vi "example_01_authorization.vi"() -> ()   [LabVIEW 2015, in "lv-dropbox.lvlib"]
uses:
  lv-dropbox.lvlib
  <vilib>/Platform/browser.llb/Open URL in Default Browser (string).vi
panel:
  in  "access_code":string
  out "challenge":string
  in  "client_id":string
  out "error":errorcluster
  out "access_token":string
  in  "app_secret":string
  in  "app_key":string
  in  "access_token":string
  in  "authorization_selection":T1(radio)
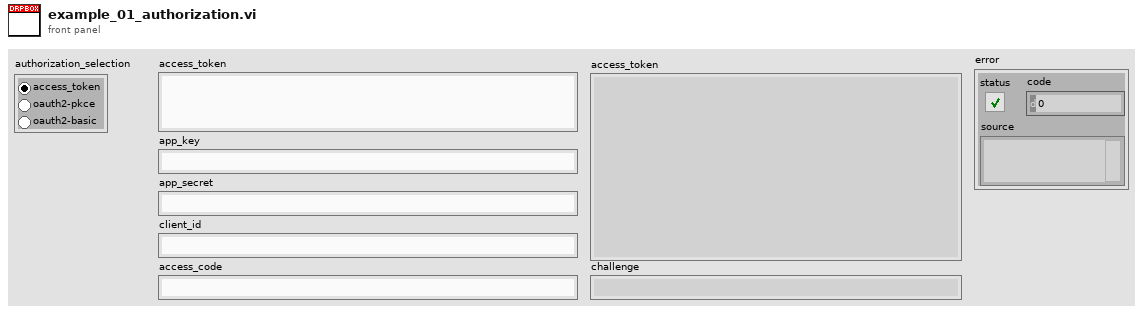
[diagram p1: front panel]
types:
  T1 = enum32{"access_token", "oauth2-pkce", "oauth2-basic"}
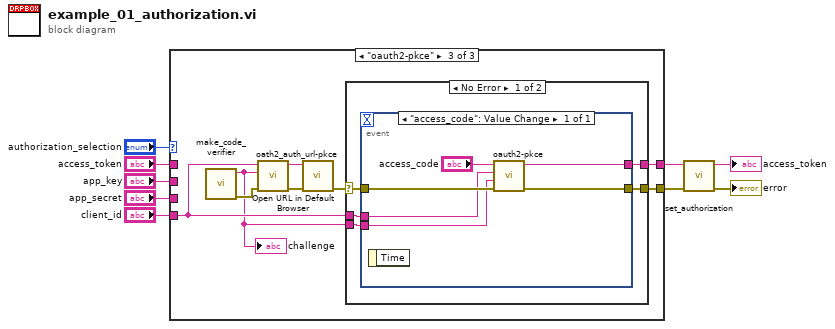
[diagram p0: block diagram]
diagram:
  n1 = case shown="\"oauth2-pkce\"" "authorization_selection" {
    tunnel: "access_token" -> [_ w9 _]
    tunnel: [_ w9 w15] -> w7
    tunnel: [_ _ w17] -> w5
    tunnel: "app_key" -> [_ _ _]
    tunnel: "app_secret" -> [_ _ _]
    tunnel: "client_id" -> [_ _ w16]
    frame Default {
    }
    frame "access_token" {
    }
    frame "oauth2-pkce" {
      n2 = call "make_code_verifier.vi"() -> ("error out"=w11:errorcluster, "code_verifier"=w10:string)  [unwired: 10 in]
      "challenge" <- w10
      n3 = call "oath2_auth_url-pkce.vi"("error in (no error)"=w11, "challenge"=w10, "client_id"=w16) -> ("error out"=w13:errorcluster, "auth_url"=w14:string)  [unwired: 7 in]
      n4 = call-poly <vilib>:"Open URL in Default Browser.vi"("error in (no error)"=w13, "URL"=w14) -> ("error out"=w12:errorcluster)  [unwired: 4 in, 1 out]
      n5 = case shown="No Error" w12 {
        selector: w12 -> [w21 w29]
        tunnel: [w22 w29] -> w17
        tunnel: w16 -> [w20 _]
        tunnel: w10 -> [w19 _]
        tunnel: [w18 _] -> w15
        frame No Error {
          n6 = event shown="[0] \"access_code\": Value Change" {
            selector: _ -> [_]
            dyn-events: _ -> [_]
            timeout: _ -> [_]
            tunnel: [w27] -> w22
            tunnel: w21 -> [w26]
            tunnel: w20 -> [w25]
            tunnel: w19 -> [w24]
            tunnel: [w23] -> w18
            event "access_code": Value Change {
              n7 = event-data() -> ()  [unwired: 1 in, 1 out]
              n8 = call "oauth2-pkce.vi"("error in (no error)"=w26, "code_verifier"=w24, "client_id"=w25, "authorization_code"="access_code") -> ("error out"=w27:errorcluster, "access_token"=w23:string)  [unwired: 6 in]
            }
          }
        }
        frame Error {
        }
      }
    }
  }
  "access_token" <- w7
  n9 = call "set_authorization.vi"("error in (no error)"=w5, "authorization"=w7) -> ("error out"=→"error":errorcluster)  [unwired: 9 in]
